vi "Untitled 4.vi"() -> ()   [LabVIEW 2021]
uses:
  Control 1.ctl
panel:
  out "Output 2":dbl(knob) scale=0.0..750.0
  in  "D":dbl(knob) scale=0.0..10.0
  in  "C":dbl(knob) scale=0.0..10.0
  in  "B":dbl(knob) scale=0.0..10.0
  in  "A":dbl(knob) min=0.0 max=10.0 step=1.0 scale=0.0..10.0
  in  "Combo Box":T1
  out "Output":dbl
  in  "Num2":dbl
  in  "num1":dbl
  # "."
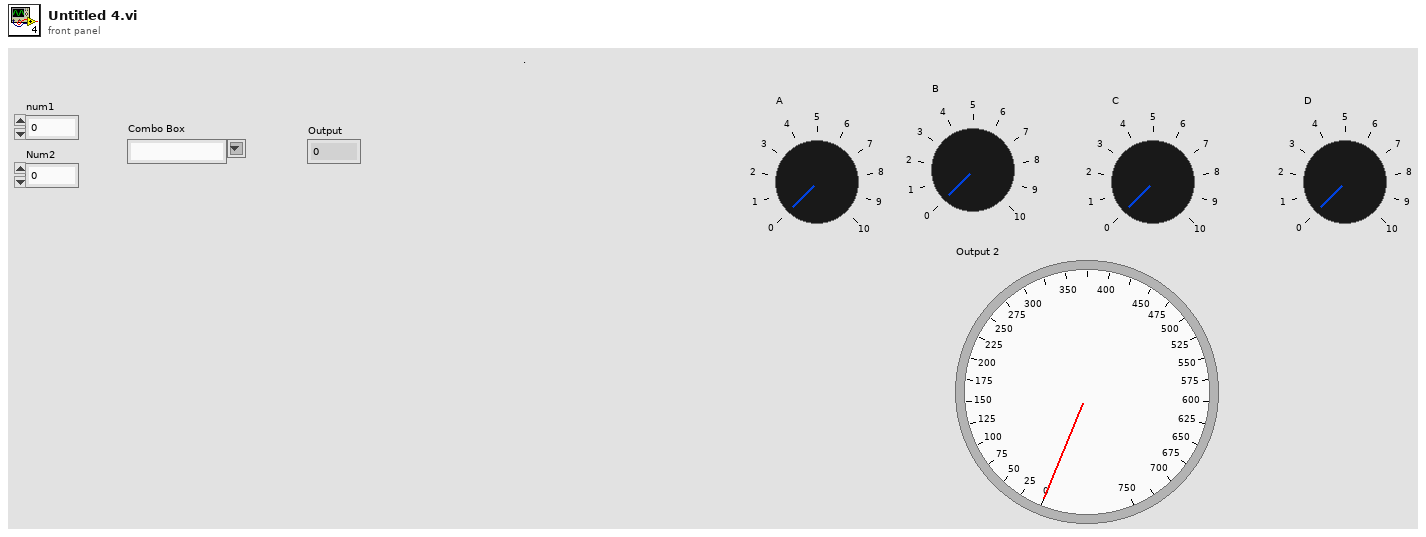
[diagram p1: front panel]
types:
  T1 = typedef "Control 1.ctl" = string
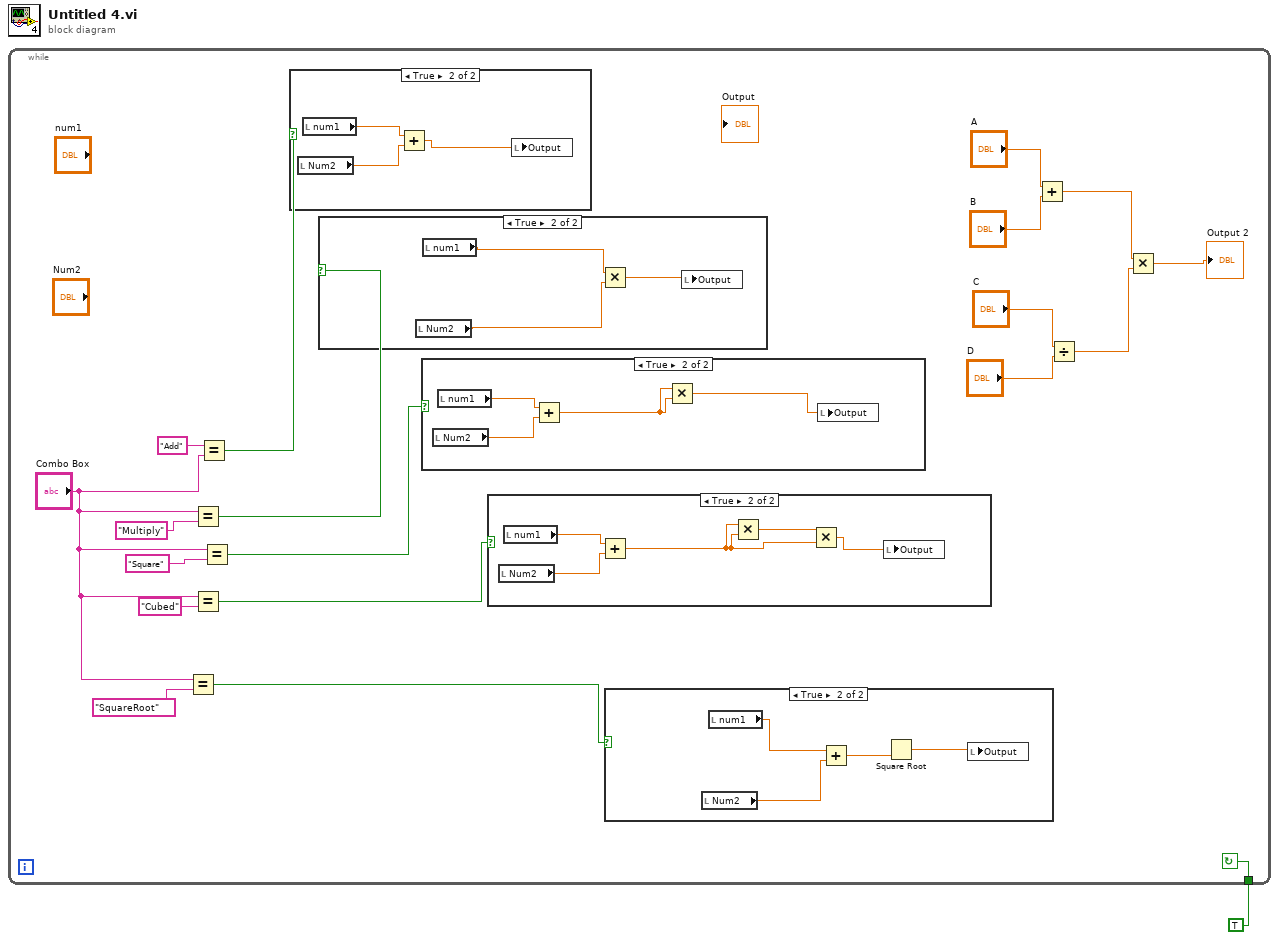
[diagram p0: block diagram]
diagram:
  n1 = while {
    tunnel: TRUE -> [w16]
    stop <- w16 continue-if-true
    n2 = Equal?(x="Combo Box", y=T1 "SquareRoot") -> (x = y?=w9:bool)
    n3 = Equal?(x="Combo Box", y="Multiply") -> (x = y?=w17:bool)
    n4 = Equal?(x="Combo Box", y="Cubed") -> (x = y?=w12:bool)
    n5 = Equal?(x="Add", y="Combo Box") -> (x = y?=w19:bool)
    n6 = Equal?(x="Combo Box", y="Square") -> (x = y?=w14:bool)
    n7 = case shown="True" w19 {
      frame False {
      }
      frame True {
        n8 = local read "Num2"() -> (w38:dbl)
        n9 = local read "num1"() -> (w39:dbl)
        n10 = Add(x=w39, y=w38) -> (x+y=w37:dbl)
        n11 = local write "Output"(w37) -> ()
      }
    }
    n12 = case shown="True" w17 {
      frame False {
      }
      frame True {
        n13 = local read "Num2"() -> (w35:dbl)
        n14 = local read "num1"() -> (w36:dbl)
        n15 = Multiply(x=w36, y=w35) -> (x*y=w34:dbl)
        n16 = local write "Output"(w34) -> ()
      }
    }
    n17 = case shown="True" w14 {
      frame False {
      }
      frame True {
        n18 = local read "Num2"() -> (w32:dbl)
        n19 = local read "num1"() -> (w33:dbl)
        n20 = Add(x=w33, y=w32) -> (x+y=w31:dbl)
        n21 = Multiply(x=w31, y=w31) -> (x*y=w30:dbl)
        n22 = local write "Output"(w30) -> ()
      }
    }
    n23 = case shown="True" w12 {
      frame False {
      }
      frame True {
        n24 = local read "Num2"() -> (w28:dbl)
        n25 = local read "num1"() -> (w29:dbl)
        n26 = Add(x=w29, y=w28) -> (x+y=w25:dbl)
        n27 = Multiply(x=w25, y=w25) -> (x*y=w27:dbl)
        n28 = Multiply(x=w27, y=w25) -> (x*y=w26:dbl)
        n29 = local write "Output"(w26) -> ()
      }
    }
    n30 = case shown="True" w9 {
      frame False {
      }
      frame True {
        n31 = local read "Num2"() -> (w23:dbl)
        n32 = local read "num1"() -> (w22:dbl)
        n33 = Add(x=w22, y=w23) -> (x+y=w21:dbl)
        n34 = Square Root(x=w21) -> (sqrt(x)=w24:dbl)
        n35 = local write "Output"(w24) -> ()
      }
    }
    n36 = Add(x="A", y="B") -> (x+y=w3:dbl)
    n37 = Divide(x="C", y="D") -> (x/y=w4:dbl)
    n38 = Multiply(x=w3, y=w4) -> (x*y=→"Output 2":dbl)
  }
